vi "Day02-04_.vi"() -> ()   [LabVIEW 2021]
panel:
  out "x+y":dbl
  in  "숫자형 4":dbl
  in  "숫자형 3":dbl
  in  "숫자형 2":dbl
  in  "숫자형":dbl
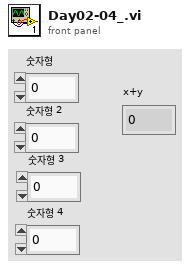
[diagram p1: front panel]
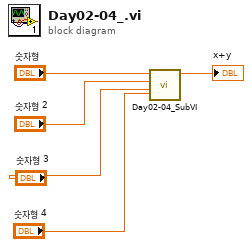
[diagram p0: block diagram]
diagram:
  n1 = call "Day02-04_SubVI.vi"("숫자형 4"="숫자형 4", "숫자형 3"="숫자형 3", "숫자형 2"="숫자형 2", "숫자형"="숫자형") -> ("x+y"=→"x+y":dbl)  [unwired: 7 in]
